vi "Whole_frame_gen_fromPark_toPark.vi"(5 "offset Y":dbl, 7 "offset X":dbl, 9 "Range":dbl=350.0, 10 "pixels":i32=256, 11 "dwell":dbl=1.0) -> (0 "Unparking _length":i32, 1 "Array Y":dbl[](array[numeric]), 2 "Array X":dbl[](array[numeric]), 4 "Base":i32=256, 6 "Bases in frame":i32)   [LabVIEW 2009]
panel:
  out "length of frame":i32
  out "Waveform Graph 4":dbl[](graph)
  out "Waveform Graph 2":dbl[](graph)
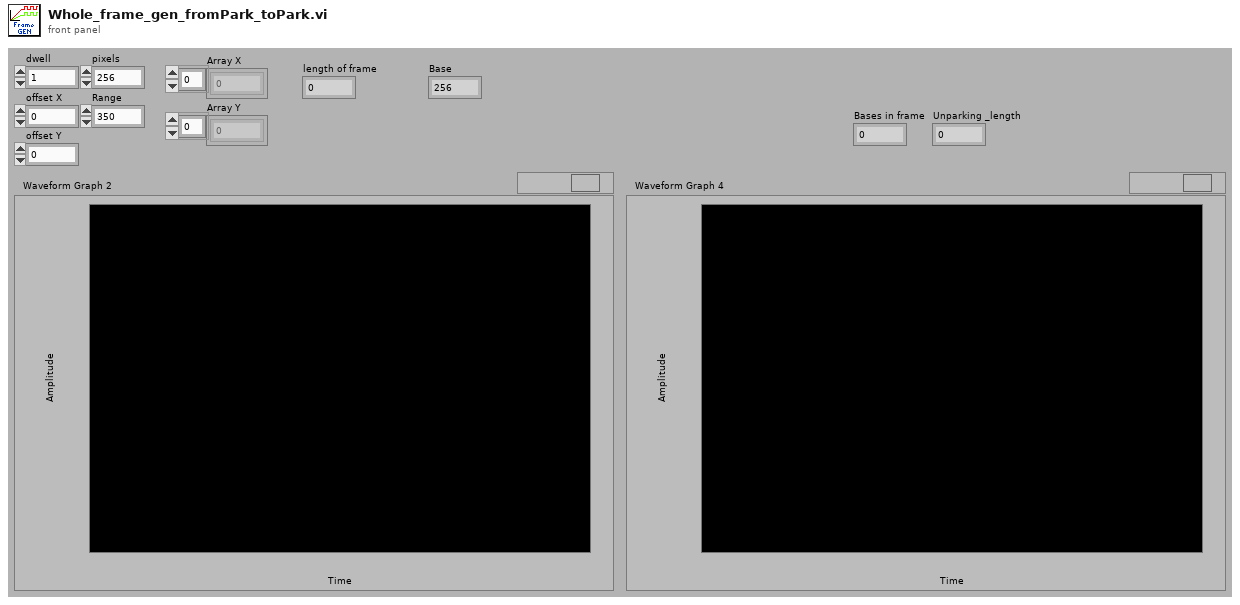
[diagram p1: front panel]
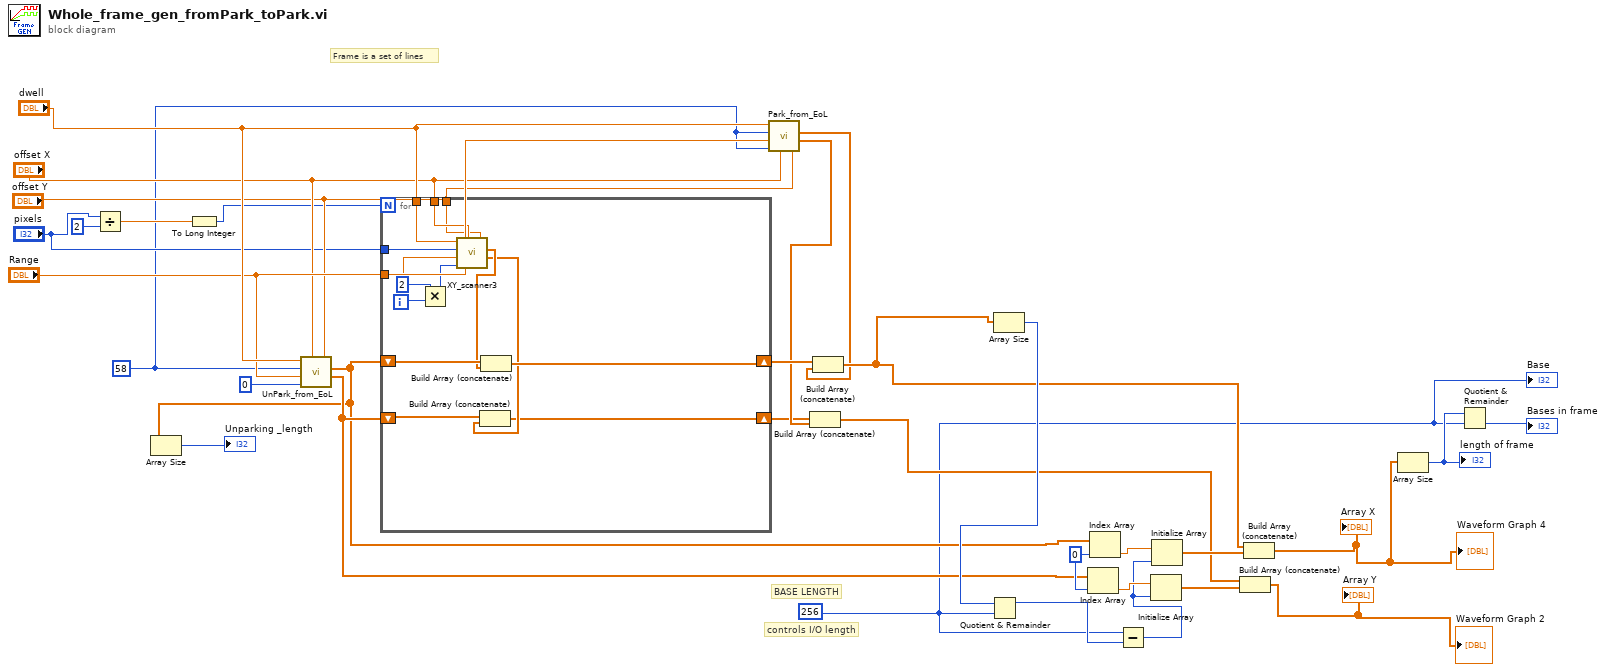
[diagram p0: block diagram]
diagram:
  w10 = 58 ("Pixels")
  w19 = 0 ("index")
  w3 = 256 ("Pixels")
  # "controls I/O length"
  # "BASE LENGTH"
  # "Frame is a set of lines"
  n1 = Divide(x="pixels", y=2) -> (x/y=w27:dbl)
  n2 = To Long Integer(number=w27) -> (32bit integer=w26:i32)
  n3 = call "UnPark_from_EoL.vi"("offset Y"="offset Y", "offset X"="offset X", "Line_start"=0, "Range"="Range", "Pixels"=w10, "dwell"="dwell") -> ("Array Y"=w14:dbl[], "Array X"=w8:dbl[])  [unwired: 1 out]
  n4 = Array Size(array=w8) -> (size(s)=→"Unparking _length":i32)
  n5 = for {
    N: w26 -> [_]
    tunnel: "dwell" -> [w46]
    tunnel: "offset X" -> [w45]
    tunnel: "Range" -> [w44]
    tunnel: "offset Y" -> [w43]
    tunnel: "pixels" -> [w42]
    shift-right: [w36] -> w23
    shift-left: w8 -> [w38]
    shift-right: [w33] -> w21
    shift-left: w14 -> [w35]
    i -> [w41]
    n6 = Multiply(x=2, y=w41) -> (x*y=w39:i32)
    n7 = call "XY_scanner3.vi"("offset Y"=w43, "offset X"=w45, "Line_start"=w39, "Range"=w44, "Pixels"=w42, "dwell"=w46) -> ("Array Y"=w34:dbl[], "Array X"=w37:dbl[])  [unwired: 2 out]
    n8 = Build Array (concatenate)(w35, w34) -> (w33:dbl[])
    n9 = Build Array (concatenate)(w38, w37) -> (w36:dbl[])
  }
  n10 = call "Park_from_EoL.vi"("offset Y"="offset Y", "offset X"="offset X", "Line_start"=w10, "Range"="Range", "Pixels"=w10, "dwell"="dwell") -> ("Array Y"=w22:dbl[], "Array X"=w1:dbl[])  [unwired: 1 in, 1 out]
  n11 = Build Array (concatenate)(w21, w22) -> (w13:dbl[])
  n12 = Build Array (concatenate)(w23, w1) -> (w12:dbl[])
  n13 = Array Size(array=w12) -> (size(s)=w15:i32)
  n14 = Quotient & Remainder(x=w15, y=w3) -> (x-y*floor(x/y)=w7:i32)  [unwired: 1 out]
  n15 = Index Array(array=w14, index=w19) -> (element=w18:dbl)
  n16 = Index Array(array=w8, index=w19) -> (element=w20:dbl)
  n17 = Subtract(x=w3, y=w7) -> (x-y=w6:i32)
  n18 = Initialize Array(w18, w6) -> (w16:dbl[])
  n19 = Initialize Array(w20, w6) -> (w17:dbl[])
  n20 = Build Array (concatenate)(w13, w16) -> (→"Waveform Graph 2" →"Array Y":dbl[])
  n21 = Build Array (concatenate)(w12, w17) -> (w9:dbl[])
  "Waveform Graph 4" <- w9
  "Array X" <- w9
  n22 = Array Size(array=w9) -> (size(s)=w5:i32)
  "length of frame" <- w5
  n23 = Quotient & Remainder(x=w5, y=w3) -> (floor(x/y)=→"Bases in frame":i32)  [unwired: 1 out]
  "Base" <- w3
